vi "Roll Up.vi"() -> ()   [LabVIEW 2015]
uses:
  RollUpStates.ctl
  Support/Global Objects.vi
panel:
  in  "DeclineTimeDecline":i32
  in  "Motor Power":dbl=0.23
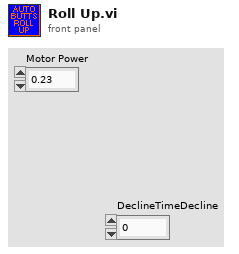
[diagram p1: front panel]
types:
  T1 = typedef "RollUpStates.ctl" = enum16{"Driving Forward", "Wait for Incline", "Stop"}
  T2 = typedef "NaxX Info.ctl" = cluster{"navX Device":T3, "Current Yaw":dbl, "Active":bool, "Current Roll":dbl}
  T3 = typedef "navX Library v2.lvlib/Z900_navX_DeviceTypeDef.ctl" = cluster{"Interface":cluster{"Protocol":T4, "Update Rate (4Hz-60Hz)":u8, "navX Open TypeDef":variant}, "Notify Packet":refnum<notifier>, "Loop VI Refnum":refnum<vi>, "Ready to Close Occurrence Refnum":refnum<k4>}
  T4 = typedef "navX Library v2.lvlib/Z900_navX_ProtocolTypeDef.ctl" = enum16{"SERIAL", "I2C", "SPI"}
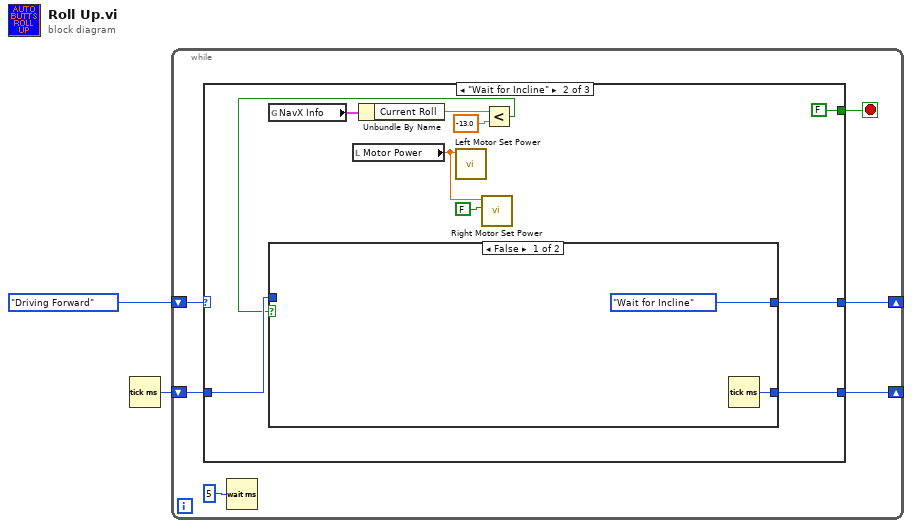
[diagram p0: block diagram]
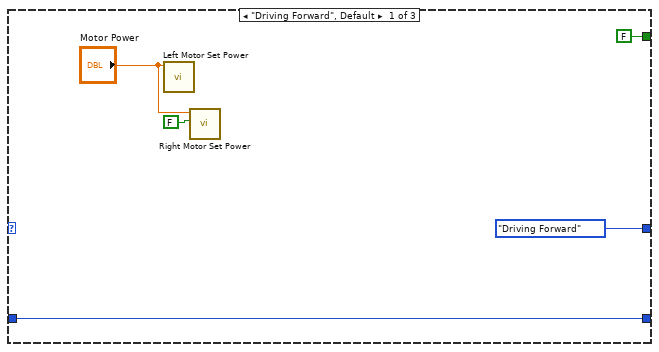
[diagram p2: hidden frame]
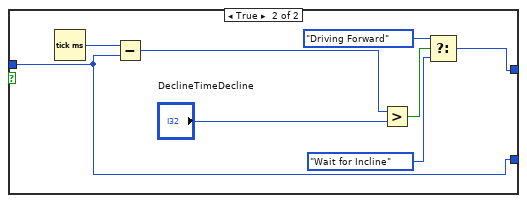
[diagram p3: hidden frame]
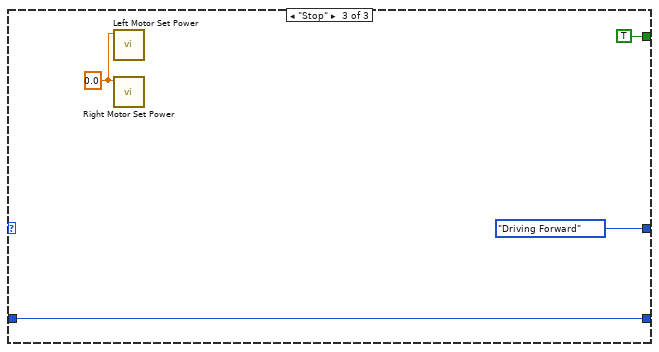
[diagram p4: hidden frame]
diagram:
  n1 = Tick Count (ms)() -> (millisecond timer value=w2:u32)
  n2 = while {
    shift-right: [w7] -> _
    shift-left: RollUpStates."Driving Forward" -> [w8]
    shift-right: [w4] -> _
    shift-left: w2 -> [w3]
    stop <- w6 stop-if-true
    n3 = case shown="\"Wait for Incline\"" w8 {
      tunnel: [RollUpStates."Driving Forward" w17 RollUpStates."Driving Forward"] -> w7
      tunnel: [FALSE FALSE TRUE] -> w6
      tunnel: [w10 w19 w35] -> w4
      tunnel: w3 -> [w10 w20 w35]
      frame "Driving Forward", Default {
        n4 = call "Left Motor Set Power.vi"("Output"="Motor Power") -> ()  [unwired: 10 in, 1 out]
        n5 = call "Right Motor Set Power.vi"("Disable Ramp"=FALSE, "Output"="Motor Power") -> ()  [unwired: 9 in, 1 out]
      }
      frame "Wait for Incline" {
        n6 = global read "Global Objects.vi" "NavX Info"() -> (w18:T2)
        n7 = local read "Motor Power"() -> (w21:dbl)
        n8 = Unbundle By Name(w18) -> ("Current Roll"=w16:dbl)
        n9 = call "Left Motor Set Power.vi"("Output"=w21) -> ()  [unwired: 10 in, 1 out]
        n10 = call "Right Motor Set Power.vi"("Disable Ramp"=FALSE, "Output"=w21) -> ()  [unwired: 9 in, 1 out]
        n11 = Less?(x=w16, y=-13.0) -> (x < y?=w14:bool)
        n12 = case shown="False" w14 {
          tunnel: [w25 w28] -> w19
          tunnel: [RollUpStates."Wait for Incline" w30] -> w17
          tunnel: w20 -> [_ w28]
          frame False {
            n13 = Tick Count (ms)() -> (millisecond timer value=w25:u32)
          }
          frame True {
            n14 = Tick Count (ms)() -> (millisecond timer value=w33:u32)
            n15 = Subtract(x=w33, y=w28) -> (x-y=w32:u32)
            n16 = Greater?(x=w32, y="DeclineTimeDecline") -> (0:w31:bool)
            n17 = Select(t=RollUpStates."Driving Forward", s=w31, f=RollUpStates."Wait for Incline") -> (s? t:f=w30:T1)
          }
        }
      }
      frame "Stop" {
        w36 = 0.0 ("Output")
        n18 = call "Left Motor Set Power.vi"("Output"=w36) -> ()  [unwired: 10 in, 1 out]
        n19 = call "Right Motor Set Power.vi"("Output"=w36) -> ()  [unwired: 10 in, 1 out]
      }
    }
    n20 = Wait (ms)(milliseconds to wait=u32 5) -> ()  [unwired: 1 out]
  }
